vi "singleActionZaberGUI.vi"() -> ()   [LabVIEW 2013]
uses:
  <instrlib>/ZaberTSeries/ZaberTSeries.lvlib
panel:
  in  "VISA resource":refnum<visa-resource-name>="COM3"
  in  "Stop VI":bool
  out "Max speed (mm):":dbl=18.0 format="%#.3g"
  out "Step size (mm):":dbl=0.49609375 format="%#.3g"
  out "Max position (mm):":dbl=151.49760546875 format="%#.3g"
  out "Current position (mm):":dbl format="%#.3g"
  in  "Position (mm)":dbl min=-151.488 max=151.498 step=0.001 format="%#.3g"
  in  "right but":bool
  in  "left but":bool
  in  "go but":bool
  in  "home but":bool
  in  "stop but":bool
  in  "radio but":enum32{"Absolute", "Relative"}(radio)
  in  "Speed (mm/s)":dbl=13.59 min=0.1 max=18.0 step=0.001 format="%.3g"
  # "Stage panel"
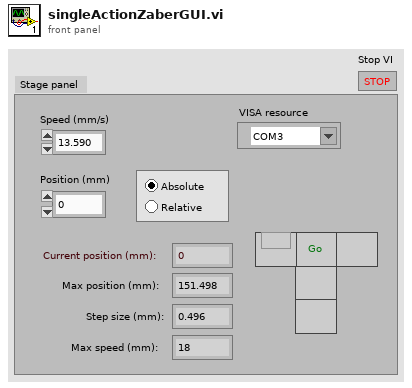
[diagram p1: front panel]
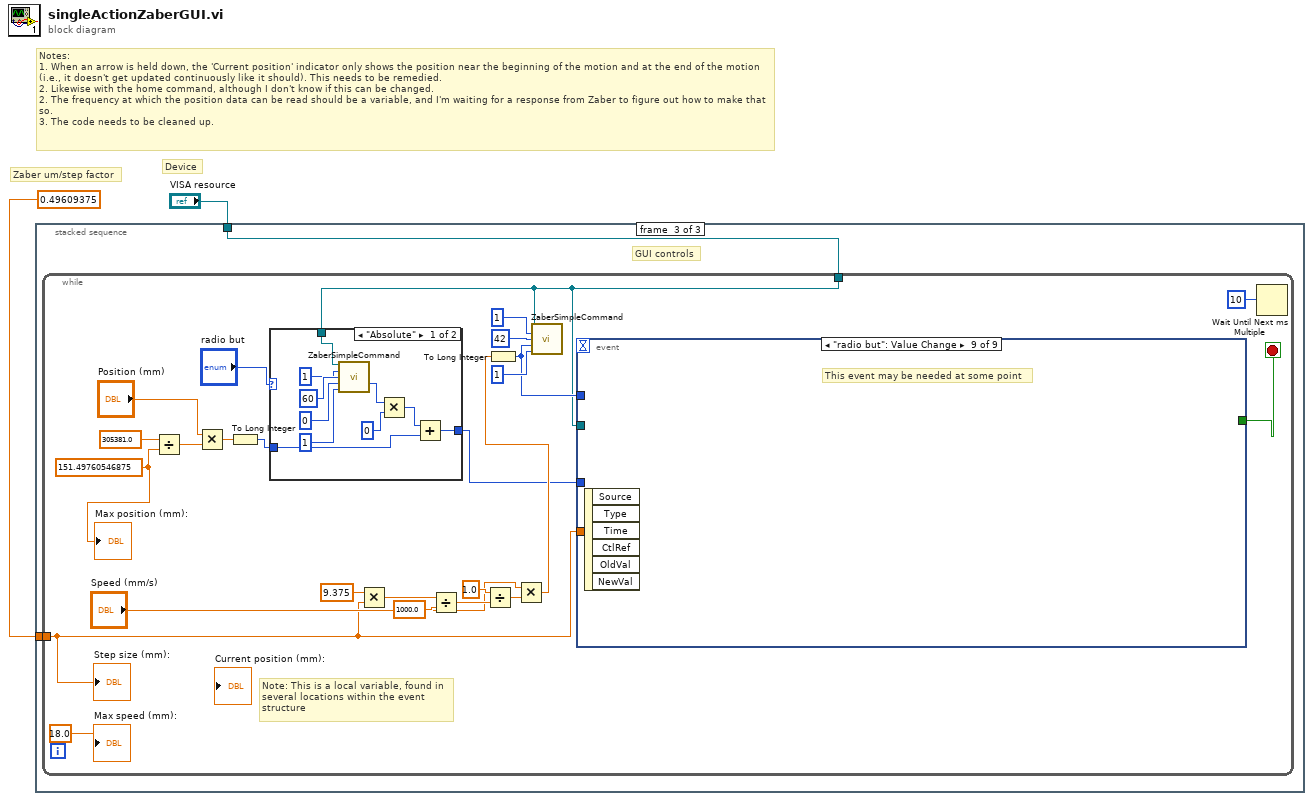
[diagram p0: block diagram]
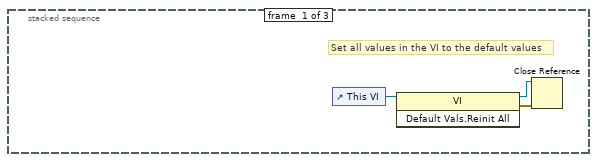
[diagram p2: hidden frame]
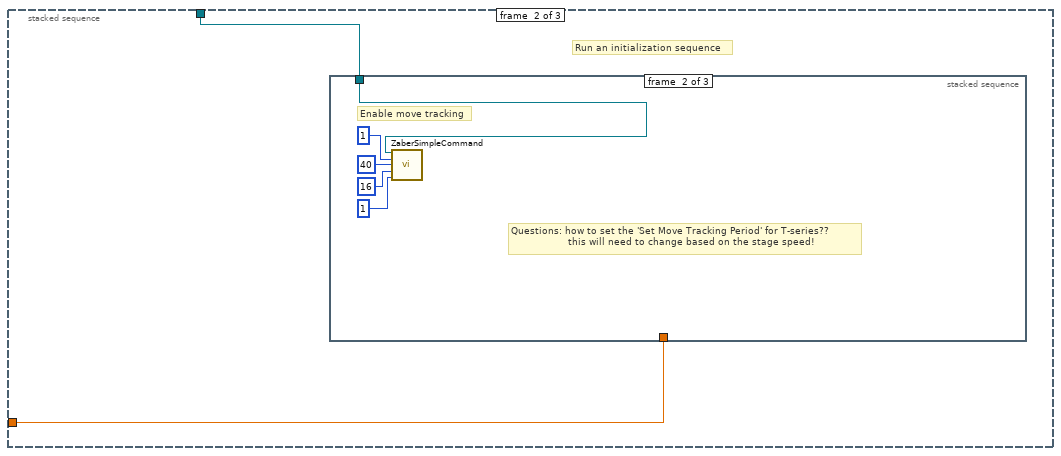
[diagram p3: hidden frame]
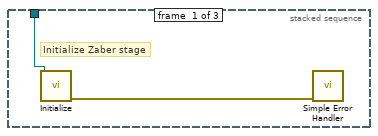
[diagram p4: hidden frame]
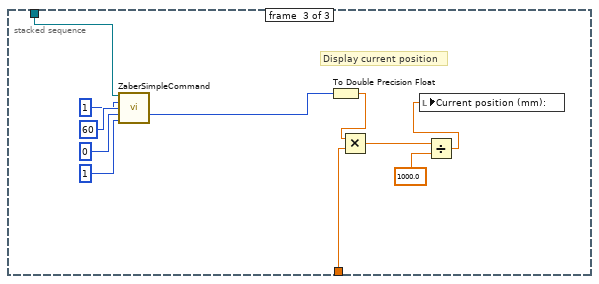
[diagram p5: hidden frame]
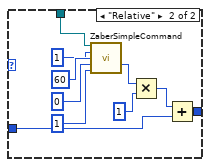
[diagram p6: hidden frame]
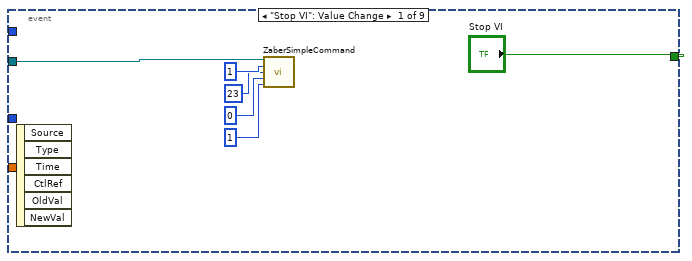
[diagram p7: hidden frame]
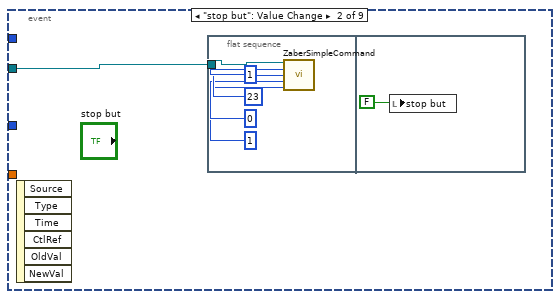
[diagram p8: hidden frame]
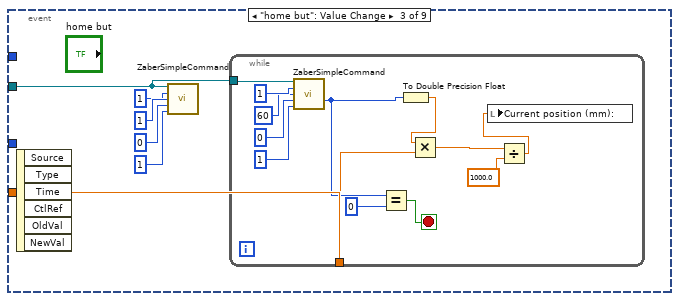
[diagram p9: hidden frame]
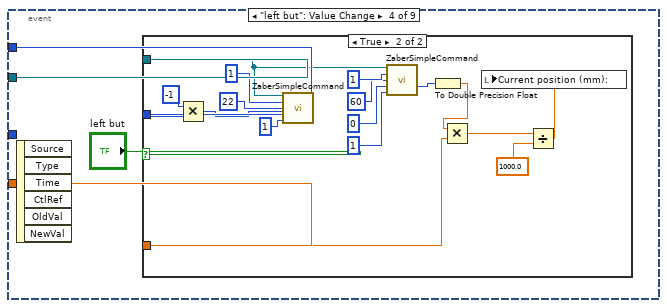
[diagram p10: hidden frame]
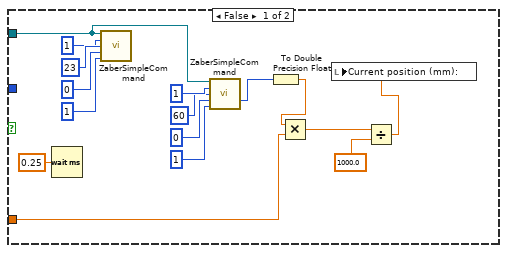
[diagram p11: hidden frame]
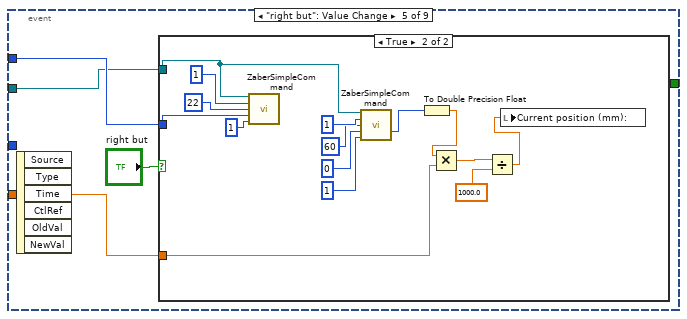
[diagram p12: hidden frame]
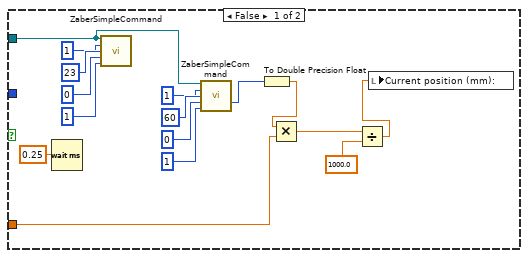
[diagram p13: hidden frame]
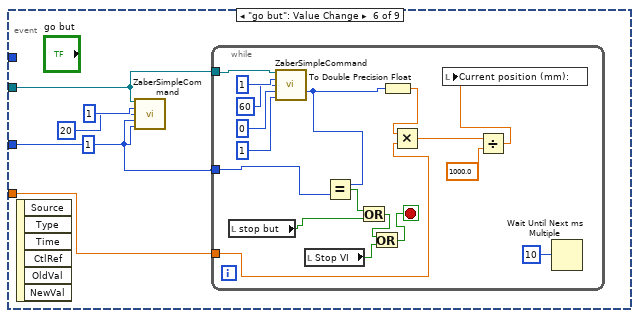
[diagram p14: hidden frame]
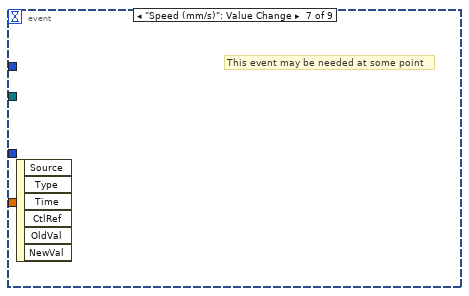
[diagram p15: hidden frame]
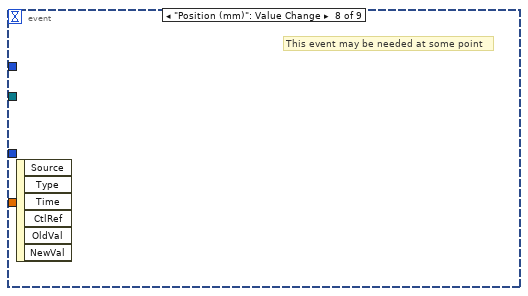
[diagram p16: hidden frame]
diagram:
  # "Notes:\n1. When an arrow is held down, the 'Current position' indicator only shows the position near the beginning of the motion and at the end of the motion (i.e., it doesn't get updated continuously like it should). This needs to be remedied.\n2. Likewise with the home command, although I don't know if this can be changed.\n2. The frequency at which the position data can be read should be a variable, and I'm waiting for a response from Zaber to figure out how to make that so.\n3. The code needs to be cleaned up."
  # "Zaber um/step factor"
  # "Device"
  n1 = stacked-sequence {
    tunnel: "VISA resource" -> [_ w7 w27]
    tunnel: 0.49609375 -> [_ w6 w26]
    frame #0 {
      # "Set all values in the VI to the default values"
      n2 = control-ref of="This VI"() -> (w3:refnum<vi>)
      n3 = invoke class="VI" method="Default Vals.Reinit All"(reference=w3) -> (reference out=w5:refnum<vi>, error out=w4:errorcluster)  [unwired: 2 in, 1 out]
      n4 = Close Reference(reference=w5, error in (no error)=w4) -> ()  [unwired: 1 out]
    }
    frame #1 {
      # "Run an initialization sequence"
      n5 = stacked-sequence {
        tunnel: w7 -> [w8 w14 w17]
        tunnel: w6 -> [_ _ w15]
        frame #0 {
          # "Initialize Zaber stage"
          n6 = call <instrlib>:"Initialize.vi"("VISA resource name"=w8) -> ("error out"=w9:errorcluster)  [unwired: 8 in, 2 out]
          n7 = call <vilib>:"Simple Error Handler.vi"("error in (no error)"=w9) -> ()  [unwired: 4 in, 5 out]
        }
        frame #1 {
          # "Enable move tracking"
          # "Questions: how to set the 'Set Move Tracking Period' for T-series??\n                   this will need to change based on the stage speed!"
          n8 = call "ZaberSimpleCommand.vi"("VISA Refnum in"=w14, "Num1"=1, "Cmd"=40, "Val"=16, "Resp num"=1) -> ()  [unwired: 8 in, 3 out]
        }
        frame #2 {
          # "Display current position"
          n9 = call "ZaberSimpleCommand.vi"("VISA Refnum in"=w17, "Num1"=1, "Cmd"=60, "Val"=0, "Resp num"=1) -> ("Val"=w23:i32)  [unwired: 8 in, 2 out]
          n10 = To Double Precision Float(number=w23) -> (double precision float=w22:dbl)
          n11 = Multiply(x=w22, y=w15) -> (x*y=w24:dbl)
          n12 = Divide(x=w24, y=1000.0) -> (x/y=w16:dbl)
          n13 = local write "Current position (mm):"(w16) -> ()
        }
      }
    }
    frame #2 {
      # "GUI controls"
      n14 = while {
        tunnel: w27 -> [w30]
        tunnel: w26 -> [w31]
        stop <- w52 stop-if-true
        w33 = 151.49760546875
        # "Note: This is a local variable, found in several locations within the event structure"
        n15 = Divide(x=305381.0, y=w33) -> (x/y=w35:dbl)
        n16 = Multiply(x="Position (mm)", y=w35) -> (x*y=w32:dbl)
        n17 = To Long Integer(number=w32) -> (32bit integer=w29:i32)
        n18 = case shown="\"Absolute\"" "radio but" {
          tunnel: w30 -> [w58 w65]
          tunnel: w29 -> [w57 w64]
          tunnel: [w53 w63] -> w28
          frame "Absolute" {
            n19 = call "ZaberSimpleCommand.vi"("VISA Refnum in"=w58, "Num1"=1, "Cmd"=60, "Val"=0, "Resp num"=1) -> ("Val"=w56:i32)  [unwired: 8 in, 2 out]
            n20 = Multiply(x=w56, y=0) -> (x*y=w54:i32)
            n21 = Add(x=w54, y=w57) -> (x+y=w53:i32)
          }
          frame "Relative" {
            n22 = call "ZaberSimpleCommand.vi"("VISA Refnum in"=w65, "Num1"=1, "Cmd"=60, "Val"=0, "Resp num"=1) -> ("Val"=w68:i32)  [unwired: 8 in, 2 out]
            n23 = Multiply(x=w68, y=1) -> (x*y=w66:i32)
            n24 = Add(x=w66, y=w64) -> (x+y=w63:i32)
          }
        }
        n25 = Multiply(x=9.375, y=w31) -> (x*y=w50:dbl)
        n26 = Divide(x=w50, y=1000.0) -> (x/y=w51:dbl)
        n27 = Divide(x=1.0, y=w51) -> (x/y=w46:dbl)
        n28 = Multiply(x="Speed (mm/s)", y=w46) -> (x*y=w45:dbl)
        n29 = To Long Integer(number=w45) -> (32bit integer=w39:i32)
        n30 = call "ZaberSimpleCommand.vi"("VISA Refnum in"=w30, "Num1"=1, "Cmd"=42, "Val"=w39, "Resp num"=1) -> ()  [unwired: 8 in, 3 out]
        n31 = event shown="[8] \"radio but\": Value Change" {
          selector: _ -> [_ _ _ _ _ _ _ _ _]
          dyn-events: _ -> [_ _ _ _ _ _ _ _ _]
          timeout: _ -> [_ _ _ _ _ _ _ _ _]
          tunnel: w30 -> [w73 w79 w87 w106 w143 w177 _ _ _]
          tunnel: ["Stop VI" _ _ _ _ _ _ _ _] -> w52
          tunnel: w39 -> [_ _ _ w107 w144 _ _ _ _]
          tunnel: w28 -> [_ _ _ _ _ w178 _ _ _]
          tunnel: w31 -> [_ _ w86 w105 w142 w179 _ _ _]
          event "Stop VI": Value Change {
            n32 = event-data() -> ()  [unwired: 1 in, 6 out]
            n33 = call "ZaberSimpleCommand.vi"("VISA Refnum in"=w73, "Num1"=1, "Cmd"=23, "Val"=0, "Resp num"=1) -> ()  [unwired: 8 in, 3 out]
          }
          event "stop but": Value Change {
            n34 = event-data() -> ()  [unwired: 1 in, 6 out]
            n35 = flat-sequence {
              tunnel: w79 -> [w80]
              frame #0 {
                n36 = call "ZaberSimpleCommand.vi"("VISA Refnum in"=w80, "Num1"=1, "Cmd"=23, "Val"=0, "Resp num"=1) -> ()  [unwired: 8 in, 3 out]
              }
              frame #1 {
                n37 = local write "stop but"(FALSE) -> ()
              }
            }
          }
          event "home but": Value Change {
            n38 = event-data() -> ()  [unwired: 1 in, 6 out]
            n39 = call "ZaberSimpleCommand.vi"("VISA Refnum in"=w87, "Num1"=1, "Cmd"=1, "Val"=0, "Resp num"=1) -> ()  [unwired: 8 in, 3 out]
            n40 = while {
              tunnel: w87 -> [w100]
              tunnel: w86 -> [w92]
              stop <- w99 stop-if-true
              n41 = call "ZaberSimpleCommand.vi"("VISA Refnum in"=w100, "Num1"=1, "Cmd"=60, "Val"=0, "Resp num"=1) -> ("Val"=w95:i32)  [unwired: 8 in, 2 out]
              n42 = Equal?(x=w95, y=0) -> (x = y?=w99:bool)
              n43 = To Double Precision Float(number=w95) -> (double precision float=w98:dbl)
              n44 = Multiply(x=w98, y=w92) -> (x*y=w96:dbl)
              n45 = Divide(x=w96, y=1000.0) -> (x/y=w94:dbl)
              n46 = local write "Current position (mm):"(w94) -> ()
            }
          }
          event "left but": Value Change {
            n47 = event-data() -> ()  [unwired: 1 in, 6 out]
            n48 = case shown="True" "left but" {
              tunnel: w106 -> [w114 w127]
              tunnel: w107 -> [_ w137]
              tunnel: w105 -> [w110 w128]
              frame False {
                n49 = Wait (ms)(milliseconds to wait=0.25) -> ()  [unwired: 1 out]
                n50 = call "ZaberSimpleCommand.vi"("VISA Refnum in"=w114, "Num1"=1, "Cmd"=23, "Val"=0, "Resp num"=1) -> ()  [unwired: 8 in, 3 out]
                n51 = call "ZaberSimpleCommand.vi"("VISA Refnum in"=w114, "Num1"=1, "Cmd"=60, "Val"=0, "Resp num"=1) -> ("Val"=w113:i32)  [unwired: 8 in, 2 out]
                n52 = To Double Precision Float(number=w113) -> (double precision float=w115:dbl)
                n53 = Multiply(x=w115, y=w110) -> (x*y=w112:dbl)
                n54 = Divide(x=w112, y=1000.0) -> (x/y=w111:dbl)
                n55 = local write "Current position (mm):"(w111) -> ()
              }
              frame True {
                n56 = Multiply(x=-1, y=w137) -> (x*y=w138:i32)
                n57 = call "ZaberSimpleCommand.vi"("VISA Refnum in"=w127, "Num1"=1, "Cmd"=22, "Val"=w138, "Resp num"=1) -> ()  [unwired: 8 in, 3 out]
                n58 = call "ZaberSimpleCommand.vi"("VISA Refnum in"=w127, "Num1"=1, "Cmd"=60, "Val"=0, "Resp num"=1) -> ("Val"=w129:i32)  [unwired: 8 in, 2 out]
                n59 = To Double Precision Float(number=w129) -> (double precision float=w131:dbl)
                n60 = Multiply(x=w131, y=w128) -> (x*y=w130:dbl)
                n61 = Divide(x=w130, y=1000.0) -> (x/y=w126:dbl)
                n62 = local write "Current position (mm):"(w126) -> ()
              }
            }
          }
          event "right but": Value Change {
            n63 = event-data() -> ()  [unwired: 1 in, 6 out]
            n64 = case shown="True" "right but" {
              tunnel: w143 -> [w149 w165]
              tunnel: w144 -> [_ w173]
              tunnel: w142 -> [w148 w164]
              frame False {
                n65 = Wait (ms)(milliseconds to wait=0.25) -> ()  [unwired: 1 out]
                n66 = call "ZaberSimpleCommand.vi"("VISA Refnum in"=w149, "Num1"=1, "Cmd"=23, "Val"=0, "Resp num"=1) -> ()  [unwired: 8 in, 3 out]
                n67 = call "ZaberSimpleCommand.vi"("VISA Refnum in"=w149, "Num1"=1, "Cmd"=60, "Val"=0, "Resp num"=1) -> ("Val"=w155:i32)  [unwired: 8 in, 2 out]
                n68 = To Double Precision Float(number=w155) -> (double precision float=w154:dbl)
                n69 = Multiply(x=w154, y=w148) -> (x*y=w156:dbl)
                n70 = Divide(x=w156, y=1000.0) -> (x/y=w147:dbl)
                n71 = local write "Current position (mm):"(w147) -> ()
              }
              frame True {
                n72 = call "ZaberSimpleCommand.vi"("VISA Refnum in"=w165, "Num1"=1, "Cmd"=22, "Val"=w173, "Resp num"=1) -> ()  [unwired: 8 in, 3 out]
                n73 = call "ZaberSimpleCommand.vi"("VISA Refnum in"=w165, "Num1"=1, "Cmd"=60, "Val"=0, "Resp num"=1) -> ("Val"=w167:i32)  [unwired: 8 in, 2 out]
                n74 = To Double Precision Float(number=w167) -> (double precision float=w168:dbl)
                n75 = Multiply(x=w168, y=w164) -> (x*y=w166:dbl)
                n76 = Divide(x=w166, y=1000.0) -> (x/y=w162:dbl)
                n77 = local write "Current position (mm):"(w162) -> ()
              }
            }
          }
          event "go but": Value Change {
            n78 = event-data() -> ()  [unwired: 1 in, 6 out]
            n79 = call "ZaberSimpleCommand.vi"("VISA Refnum in"=w177, "Num1"=1, "Cmd"=20, "Val"=w178, "Resp num"=1) -> ()  [unwired: 8 in, 3 out]
            n80 = while {
              tunnel: w177 -> [w185]
              tunnel: w178 -> [w196]
              tunnel: w179 -> [w186]
              stop <- w187 stop-if-true
              n81 = local read "stop but"() -> (w184:bool)
              n82 = call "ZaberSimpleCommand.vi"("VISA Refnum in"=w185, "Num1"=1, "Cmd"=60, "Val"=0, "Resp num"=1) -> ("Val"=w192:i32)  [unwired: 8 in, 2 out]
              n83 = local read "Stop VI"() -> (w189:bool)
              n84 = Equal?(x=w192, y=w196) -> (x = y?=w190:bool)
              n85 = Or(x=w190, y=w184) -> (x .or. y?=w188:bool)
              n86 = Or(x=w188, y=w189) -> (x .or. y?=w187:bool)
              n87 = To Double Precision Float(number=w192) -> (double precision float=w195:dbl)
              n88 = Multiply(x=w195, y=w186) -> (x*y=w193:dbl)
              n89 = Divide(x=w193, y=1000.0) -> (x/y=w191:dbl)
              n90 = local write "Current position (mm):"(w191) -> ()
              n91 = Wait Until Next ms Multiple(millisecond multiple=10) -> ()  [unwired: 1 out]
            }
          }
          event "Speed (mm/s)": Value Change {
            # "This event may be needed at some point"
            n92 = event-data() -> ()  [unwired: 1 in, 6 out]
          }
          event "Position (mm)": Value Change {
            # "This event may be needed at some point"
            n93 = event-data() -> ()  [unwired: 1 in, 6 out]
          }
          event "radio but": Value Change {
            # "This event may be needed at some point"
            n94 = event-data() -> ()  [unwired: 1 in, 6 out]
          }
        }
        n95 = Wait Until Next ms Multiple(millisecond multiple=10) -> ()  [unwired: 1 out]
        "Max position (mm):" <- w33
        "Step size (mm):" <- w31
        "Max speed (mm):" <- 18.0
      }
    }
  }
